vi "IR1000HzcamerarReadringblockfutur_SD.vi"(0 "Nombre d'acquisitions":i32) -> (1 "temps d'acqu ms":u32, 2 "Data THz1000Hz":u32[][](graph) caption="Data Values", 3 "Nombre de spectres":i32)   [LabVIEW 2015]
panel:
  # "!!! Ne jamais lancer le VI si le VI d'initialisation n'a pas été lancé!"
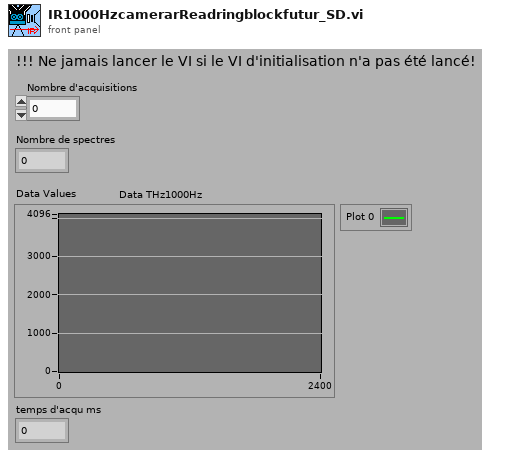
[diagram p1: front panel]
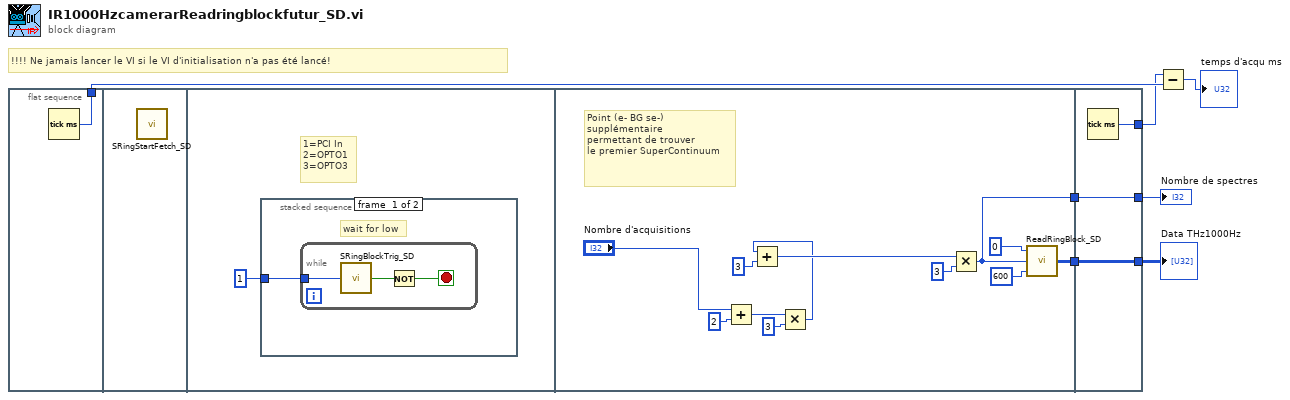
[diagram p0: block diagram]
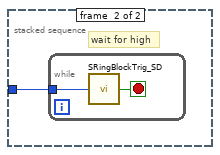
[diagram p2: hidden frame]
diagram:
  # "!!!! Ne jamais lancer le VI si le VI d'initialisation n'a pas été lancé!"
  n1 = flat-sequence {
    tunnel: [w8] -> w4
    tunnel: [w27] -> w7
    tunnel: [w22] -> w6
    tunnel: w7 -> [w29]
    tunnel: w6 -> [w30]
    tunnel: [w31] -> w3
    tunnel: [w30] -> w2
    tunnel: [w29] -> w1
    frame #0 {
      n2 = Tick Count (ms)() -> (millisecond timer value=w8:u32)
    }
    frame #1 {
      n3 = call "SRingStartFetch_SD.vi"() -> ()  [unwired: 2 in]
    }
    frame #2 {
      # "1=PCI In\n2=OPTO1\n3=OPTO3"
      n4 = stacked-sequence {
        tunnel: u8 1 -> [w10 w14]
        frame #0 {
          # "wait for low"
          n5 = while {
            tunnel: w10 -> [w11]
            stop <- w13 stop-if-true
            n6 = call "SRingBlockTrig_SD.vi"("channel 1, 2 or 3"=w11) -> ("Boolesch"=w12:bool)
            n7 = Not(x=w12) -> (.not. x?=w13:bool)
          }
        }
        frame #1 {
          # "wait for high"
          n8 = while {
            tunnel: w14 -> [w15]
            stop <- w16 stop-if-true
            n9 = call "SRingBlockTrig_SD.vi"("channel 1, 2 or 3"=w15) -> ("Boolesch"=w16:bool)
          }
        }
      }
    }
    frame #3 {
      # "Point (e- BG se-) \nsupplémentaire\npermettant de trouver \nle premier SuperContinuum"
      n10 = Add(x="Nombre d'acquisitions", y=2) -> (x+y=w21:i32)
      n11 = Multiply(x=w21, y=3) -> (x*y=w17:i32)
      n12 = Add(x=w17, y=3) -> (x+y=w24:i32)
      n13 = Multiply(x=w24, y=3 ("Nombre de pulse par acqu")) -> (x*y=w22:i32)
      n14 = call "ReadRingBlock_SD.vi"("pixel"=u32 600, "stop"=w22, "start"=0 ("stop")) -> ("Data Values"=w27:u32[][])
    }
    frame #4 {
      n15 = Tick Count (ms)() -> (millisecond timer value=w31:u32)
    }
  }
  n16 = Subtract(x=w3, y=w4) -> (x-y=→"temps d'acqu ms":u32)
  "Data THz1000Hz" <- w1
  "Nombre de spectres" <- w2
